vi "Tree Create Measurement Item.vi"(8 "error in (no error)":errorcluster, 10 "New Text Value":string, 11 "TreeControl in":refnum<vi>) -> (0 "error out":errorcluster, 2 "Created Tag":string, 3 "TreeControl out":refnum<vi>)   [LabVIEW 2019]
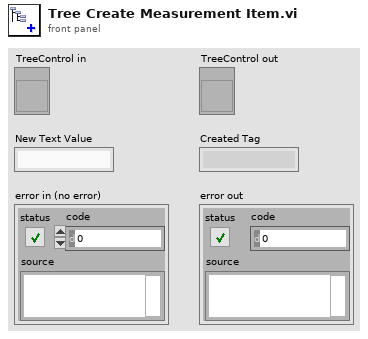
[diagram p1: front panel]
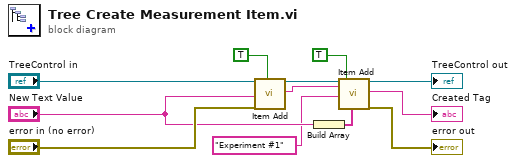
[diagram p0: block diagram]
diagram:
  n1 = call <instrlib>:"Item Add.vi"("Tree Reference In"="TreeControl in", "New Text Value"="New Text Value", "error in (no error)"="error in (no error)", "Make Top Level Item"=TRUE) -> ("Tree Reference Out"=w2:refnum<vi>, "Created Tag"=w3:string)  [unwired: 13 in, 1 out]
  n2 = Build Array("New Text Value") -> (w8:string[])
  n3 = call <instrlib>:"Item Add.vi"("Tree Reference In"=w2, "Parent Tag (Current)"=w3, "New Text Value"="Experiment #1", "Child Only?"=TRUE, "Column Text{#1 and greater}(empty)"=w8) -> ("Tree Reference Out"=→"TreeControl out":refnum<vi>, "Created Tag"=→"Created Tag":string, "error out"=→"error out":errorcluster)  [unwired: 12 in]
